vi "svacg Create Log Scale Linear Interpolated Specifications.vi"(6 "Log Specs":bool, 8 "error in (no error)":errorcluster, 9 "x0":dbl=100.0 format="%.2f", 10 "dx":dbl=100.0 format="%.2f", 11 "raw specifications":cluster{"X-specs":dbl[], "Y-specs":dbl[]} {"Y-specs" format="%.2p"; "X-specs" format="%.2p"}) -> (0 "error out":errorcluster, 1 "x0 out":dbl=100.0 format="%.2f", 2 "dx out":dbl=100.0 format="%.2f", 3 "XY pairs output":cluster{"X-data":dbl[], "Y-data":dbl[]} {"Y-data" format="%0.2f"; "X-data" format="%0.2f"})   [LabVIEW 2017]
panel:
  out "x0-dt-Y output":cluster{"x0":dbl, "dX":dbl, "Y-data":dbl[]} {"Y-data" format="%0.2f"; "dX" format="%0.2f"; "x0" format="%0.2f"}
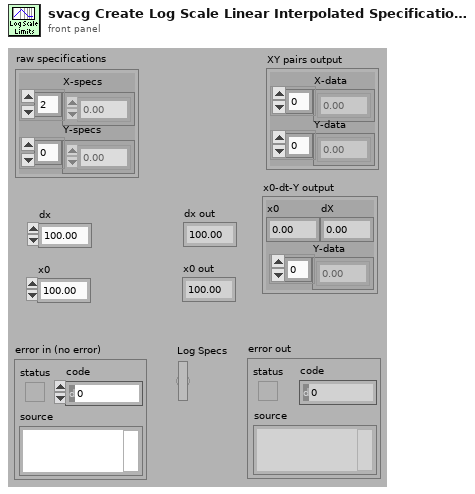
[diagram p1: front panel]
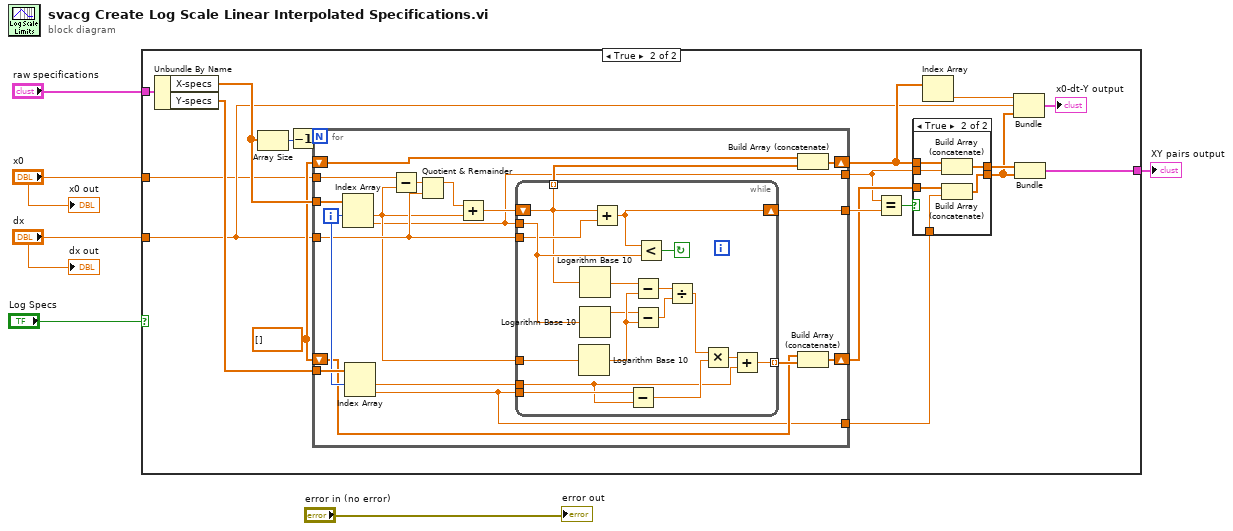
[diagram p0: block diagram]
diagram:
  n1 = case shown="True" "Log Specs" {
    tunnel: [w7 w26] -> w6
    tunnel: "raw specifications" -> [w7 w23]
    tunnel: "dx" -> [_ w9]
    tunnel: "x0" -> [_ w8]
    frame False {
    }
    frame True {
      w18 = dbl[] []
      n2 = Unbundle By Name(w23) -> ("X-specs"=w21:dbl[], "Y-specs"=w22:dbl[])
      n3 = Array Size(array=w21) -> (size(s)=w20:i32)
      n4 = Decrement(x=w20) -> (x-1=w19:i32)
      n5 = for {
        N: w19 -> [_]
        tunnel: w21 -> [w53]
        tunnel: w22 -> [w52]
        shift-right: [w47] -> w13
        shift-left: w18 -> [w48]
        tunnel: w9 -> [w42]
        shift-right: [w44] -> w15
        shift-left: w18 -> [w45]
        tunnel: w8 -> [w38]
        tunnel: [w37] -> w17
        tunnel: [w36] -> w11
        tunnel: [w35] -> w10
        i -> [w51]
        n6 = Index Array(array=w53, index #1=w51) -> (element #1=w39:dbl, element #2=w36:dbl)  [unwired: 1 in]
        n7 = Index Array(array=w52, index #1=w51) -> (element #1=w50:dbl, element #2=w35:dbl)  [unwired: 1 in]
        n8 = Subtract(x=w38, y=w39) -> (x-y=w43:dbl)
        n9 = Quotient & Remainder(x=w43, y=w42) -> (x-y*floor(x/y)=w41:dbl)  [unwired: 1 out]
        n10 = Add(x=w41, y=w39) -> (x+y=w40:dbl)
        n11 = while {
          tunnel: w36 -> [w70]
          shift-right: [w58] -> w37
          shift-left: w40 -> [w57]
          tunnel: w39 -> [w69]
          tunnel: w35 -> [w65]
          tunnel: w50 -> [w54]
          tunnel: [w61] -> w49 mode=indexing
          tunnel: w42 -> [w60]
          tunnel: [w57] -> w46 mode=indexing
          stop <- w59 continue-if-true
          n12 = Logarithm Base 10(1:w69) -> (0:w67:dbl)
          n13 = Logarithm Base 10(1:w57) -> (0:w56:dbl)
          n14 = Logarithm Base 10(1:w70) -> (0:w55:dbl)
          n15 = Add(x=w57, y=w60) -> (x+y=w58:dbl)
          n16 = Subtract(x=w65, y=w54) -> (x-y=w63:dbl)
          n17 = Subtract(x=w56, y=w67) -> (x-y=w68:dbl)
          n18 = Subtract(x=w55, y=w67) -> (x-y=w66:dbl)
          n19 = Less?(x=w58, y=w70) -> (x < y?=w59:bool)
          n20 = Divide(x=w68, y=w66) -> (x/y=w64:dbl)
          n21 = Multiply(x=w64, y=w63) -> (x*y=w62:dbl)
          n22 = Add(x=w62, y=w54) -> (x+y=w61:dbl)
        }
        n23 = Build Array (concatenate)(w45, w46) -> (w44:dbl[])
        n24 = Build Array (concatenate)(w48, w49) -> (w47:dbl[])
      }
      n25 = Equal?(x=w11, y=w17) -> (x = y?=w16:bool)
      n26 = case shown="True" w16 {
        tunnel: [w28 w34] -> w14
        tunnel: w15 -> [w28 w33]
        tunnel: w13 -> [w27 w31]
        tunnel: [w27 w32] -> w12
        tunnel: w11 -> [_ w30]
        tunnel: w10 -> [_ w29]
        frame False {
        }
        frame True {
          n27 = Build Array (concatenate)(w33, w30) -> (w34:dbl[])
          n28 = Build Array (concatenate)(w31, w29) -> (w32:dbl[])
        }
      }
      n29 = Index Array(array=w15) -> (element=w25:dbl)  [unwired: 1 in]
      n30 = Bundle(w25, "dx"=w9, w12) -> (→"x0-dt-Y output":cluster{dbl, "dx":dbl, dbl[]})  [unwired: 1 in]
      n31 = Bundle(w14, w12) -> (w26:cluster{dbl[], dbl[]})  [unwired: 1 in]
    }
  }
  "XY pairs output" <- w6
  "error out" <- "error in (no error)"
  "dx out" <- "dx"
  "x0 out" <- "x0"
